vi "Is Micron sm130.vi"(8 "error in (no error)":errorcluster, 9 "Timeout":u32=10000, 10 "ID Query (True)":bool=TRUE, 11 "VISA resource name":refnum<visa-resource-name>) -> (0 "error out":errorcluster, 2 "Micron sm130":bool, 3 "VISA resource name out":refnum<visa-resource-name>)   [LabVIEW 2024]
doc: "Establishes communication with the instrument and optionally performs an instrument identification query and/or an instrument reset. It also places the instrument in a default state needed for other instrument driver operations. Therefore, call this VI before calling other instrument driver VIs for this instrument. Generally, you need to call the Initialize VI only once at the beginning of an application."
panel:
  # "(c) 2009 - 2012 National Instruments.  ALL RIGHTS RESERVED."
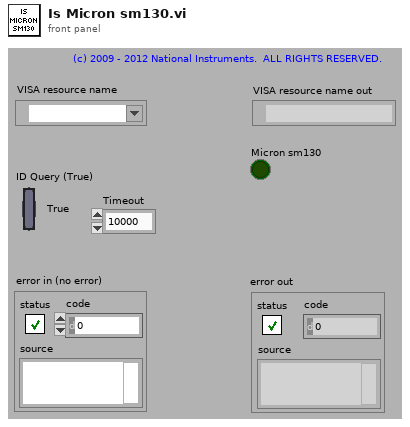
[diagram p1: front panel]
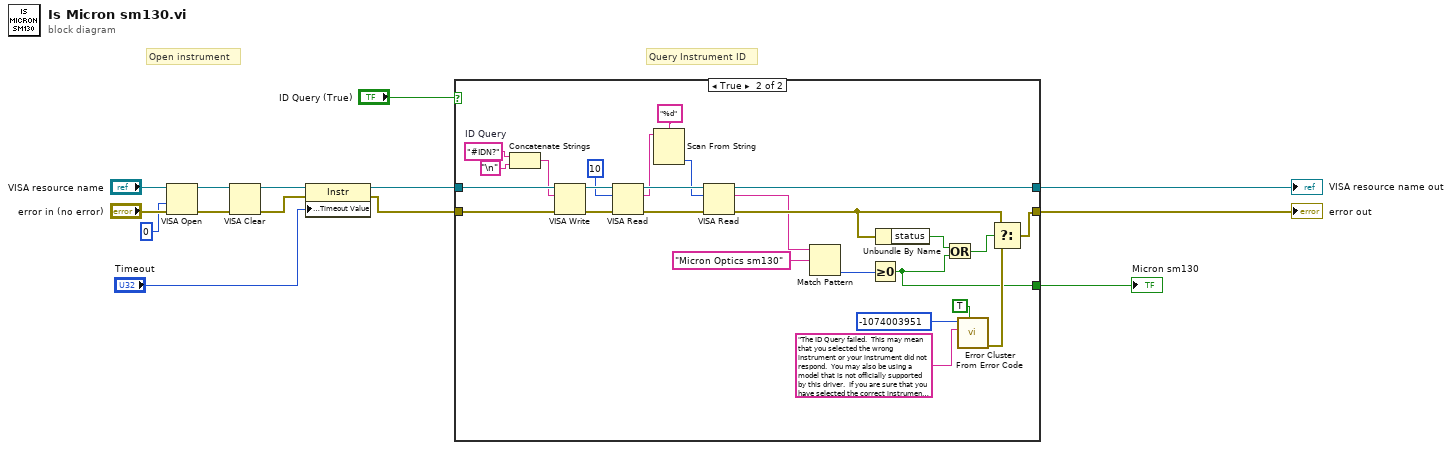
[diagram p0: block diagram]
diagram:
  # "Query Instrument ID"
  # "Open instrument"
  n1 = VISA Open(access mode=u32 0, error in (no error)="error in (no error)", VISA resource name="VISA resource name") -> (VISA resource name=w9:refnum<visa-resource-name>, error out=w8:errorcluster)  [unwired: 2 in]
  n2 = VISA Clear(VISA resource name=w9, error in (no error)=w8) -> (VISA resource name out=w7:refnum<visa-resource-name>, error out=w6:errorcluster)
  n3 = property class="Instr"(reference=w7, error in=w6, "General Settings:Timeout Value"="Timeout") -> (reference out=w5:refnum<visa-resource-name>, error out=w4:errorcluster)
  n4 = case shown="True" "ID Query (True)" {
    tunnel: [w15 w42] -> w2
    tunnel: [w16 w26] -> w3
    tunnel: w5 -> [w16 w40]
    tunnel: w4 -> [w15 w41]
    tunnel: [_ w17] -> w1
    frame False {
    }
    frame True {
      w20 = "#IDN?"  # ID Query
      n5 = Concatenate Strings(w20, "\n") -> (w18:string)
      n6 = VISA Write(VISA resource name=w40, write buffer=w18, error in (no error)=w41) -> (VISA resource name out=w39:refnum<visa-resource-name>, error out=w38:errorcluster)  [unwired: 1 out]
      n7 = VISA Read(VISA resource name=w39, byte count=u32 10, error in (no error)=w38) -> (VISA resource name out=w28:refnum<visa-resource-name>, read buffer=w24:string, error out=w27:errorcluster)  [unwired: 1 out]
      n8 = Scan From String(format string="%d", input string=w24) -> (output 1=w23:i32)  [unwired: 3 in, 3 out]
      n9 = VISA Read(VISA resource name=w28, byte count=w23, error in (no error)=w27) -> (VISA resource name out=w26:refnum<visa-resource-name>, read buffer=w21:string, error out=w25:errorcluster)  [unwired: 1 out]
      n10 = Match Pattern(string=w21, regular expression="Micron Optics sm130") -> (offset past match=w31:i32)  [unwired: 1 in, 3 out]
      n11 = Greater Or Equal To 0?(x=w31) -> (x >= 0?=w17:bool)
      n12 = Unbundle By Name(w25) -> ("status"=w30:bool)
      n13 = Or(x=w30, y=w17) -> (x .or. y?=w29:bool)
      n14 = call <vilib>:"Error Cluster From Error Code.vi"("show call chain? (False)"=TRUE, "error message (\"\")"="The ID Query failed.  This may mean that you selected the wrong instrument or your instrument did not respond.  You may also be using a model that is not officially supported by this driver.  If you are sure that you have selected the correct instrument and it is responding, try disabling the ID Query." ("Source (VI Name)"), "error code (0)"=-1074003951 ("Code")) -> ("error out"=w35:errorcluster)  [unwired: 6 in]
      n15 = Select(t=w25, s=w29, f=w35) -> (s? t:f=w42:errorcluster)
    }
  }
  "VISA resource name out" <- w3
  "error out" <- w2
  "Micron sm130" <- w1
